vi "Load Config.vi"(6 "Constants":refnum<class "Sequence Constants.lvclass">, 8 "error in (no error)":refnum<class "MultiErrors.lvclass">, 10 "Config Element":refnum<class "Config Element.lvclass">, 11 "SeqRunning Condition Config in":refnum<class "SeqRunning Condition Config.lvclass">) -> (0 "error out":refnum<class "MultiErrors.lvclass">, 3 "SeqRunning Condition Config out":refnum<class "SeqRunning Condition Config.lvclass">)   [LabVIEW 2020, in "VolatusSeqConfig.lvlib" / "SeqRunning Condition Config.lvclass"]
uses:
  SeqRunning Condition Config.lvclass
  VolatusErrorUtilities/MultiErrors/MultiErrors.lvclass
  lv-cdm/CDM-Config/Config Element/Config Element.lvclass
  SeqRunning Condition Config.lvclass/SeqRunning Condition Config.ctl
  Sequence Constants/Sequence Constants.lvclass
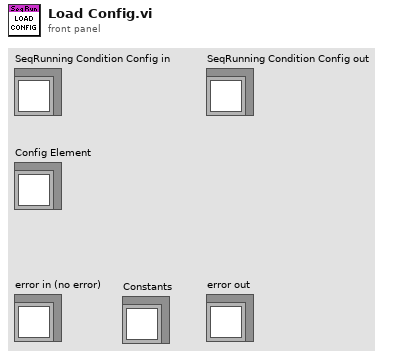
[diagram p1: front panel]
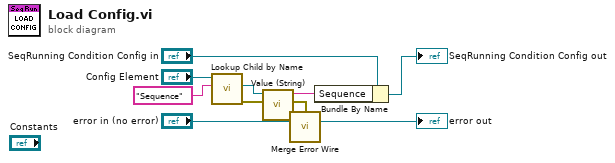
[diagram p0: block diagram]
diagram:
  n1 = call "Lookup Child by Name.vi"("Name"="Sequence", "Config Element in"="Config Element") -> ("error out"=w6:errorcluster, "Child"=w5:refnum<class "Config Element.lvclass">)  [unwired: 6 in, 2 out]
  n2 = call "Value (String).vi"("error in (no error)"=w6, "Config Element in"=w5) -> ("error out"=w3:errorcluster, "String Value"=w1:string)  [unwired: 8 in]
  n3 = call "Merge Error Wire.vi"("error in (no error)"=w3, "MultiErrors in"="error in (no error)") -> ("MultiErrors out"=→"error out":refnum<class "MultiErrors.lvclass">)  [unwired: 13 in]
  n4 = Bundle By Name(cluster="SeqRunning Condition Config in", "Sequence"=w1) -> (→"SeqRunning Condition Config out":refnum<class "SeqRunning Condition Config.lvclass">)
